vi "Waveform output.vi"(11 "Galvo signal":u32) -> ()   [LabVIEW 2015]
uses:
  <vilib>/rvi/Emulation/niFpgaSctlEmulationGetInTimedLoop.vi
  OpenScan Labview code_20170126/Global_Sample per Frame.vi
  <vilib>/rvi/Emulation/niFpgaProcessEmulError.vi
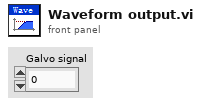
[diagram p1: front panel]
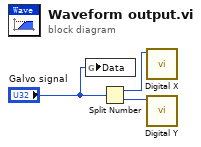
[diagram p0: block diagram]
diagram:
  n1 = global write "Global_Sample per Frame.vi" "Data"("Galvo signal") -> ()
  n2 = Split Number(x="Galvo signal") -> (hi(x)=w3:u16, lo(x)=w2:u16)
  n3 = call "Digital X.vi"("数值"=w3) -> ()  [unwired: 11 in]
  n4 = call "Digital Y.vi"("数值"=w2) -> ()  [unwired: 11 in]
